vi "TestConfig.vi"(8 "error in":errorcluster {"code" format="Error %.0f"}, 11 "MainFGV_data":T1) -> (0 "error out":errorcluster {"code" format="Error %.0f"}, 3 "MainFGV_data out":T1)   [LabVIEW 2016]
uses:
  StrainGauge/SG_data.ctl
  CurrentMeter/CM_data.ctl
  CurrentMeter/CM_SerialNumber.ctl
  MainFGV_data.ctl
panel:
  in  "OK":bool
  in  "Cancelar":bool
  in  "OpenConfig":bool caption="Abrir\nconfiguração"
  in  "SaveConfig":bool caption="Salvar\nconfiguração"
  in  "CM_config":T2[](array[typedef])=[{"Serial"=enum."274124", "Coordenada X"=0.0, "Coordenada Y"=0.0, "ID"="CH 1", "active"=TRUE}, {"Serial"=enum."274125", "Coordenada X"=0.0, "Coordenada Y"=0.0, "ID"="CH 2", "active"=TRUE}, {"Serial"=enum."274126", "Coordenada X"=0.0, "Coordenada Y"=0.0, "ID"="CH 3", "active"=TRUE}, {"Serial"=enum."274127", "Coordenada X"=0.0, "Coordenada Y"=0.0, "ID"="CH 4", "active"=TRUE}, {"Serial"=enum."274128", "Coordenada X"=0.0, "Coordenada Y"=0.0, "ID"="CH 5", "active"=TRUE}]
  in  "SG_config":T4[](array[typedef])=[{"ID"="CH 1", "Sensibilidade"=2.0, "Descrição"="Extensômetro na grade", "active"=TRUE}, {"ID"="CH 2", "Sensibilidade"=2.0, "Descrição"="Extensômetro na grade", "active"=TRUE}, {"ID"="CH 3", "Sensibilidade"=2.0, "Descrição"="Extensômetro na grade", "active"=TRUE}, {"ID"="CH 4", "Sensibilidade"=2.0, "Descrição"="Extensômetro na grade", "active"=TRUE}, {"ID"="CH 5", "Sensibilidade"=2.0, "Descrição"="Extensômetro na grade", "active"=TRUE}, {"ID"="CH 6", "Sensibilidade"=2.0, "Descrição"="Extensômetro na grade", "active"=TRUE}, {"ID"="CH 7", "Sensibilidade"=2.0, "Descrição"="Extensômetro na grade", "active"=TRUE}, {"ID"="CH 8", "Sensibilidade"=2.0, "Descrição"="Extensômetro na grade", "active"=TRUE}, {"ID"="CH 9", "Sensibilidade"=2.0, "Descrição"="Extensômetro na grade", "active"=TRUE}, {"ID"="CH 10", "Sensibilidade"=2.0, "Descrição"="Extensômetro na grade", "active"=TRUE}, {"ID"="CH 11", "Sensibilidade"=2.0, "Descrição"="Extensômetro na grade", "active"=TRUE}, {"ID"="CH 12", "Sensibilidade"=2.0, "Descrição"="Extensômetro na grade", "active"=TRUE}, {"ID"="CH 13", "Sensibilidade"=2.0, "Descrição"="Extensômetro na grade", "active"=TRUE}, {"ID"="CH 14", "Sensibilidade"=2.0, "Descrição"="Extensômetro na grade", "active"=TRUE}, {"ID"="CH 15", "Sensibilidade"=2.0, "Descrição"="Extensômetro na grade", "active"=TRUE}, {"ID"="CH 16", "Sensibilidade"=2.0, "Descrição"="Extensômetro na grade", "active"=TRUE}, {"ID"="CH 17", "Sensibilidade"=2.0, "Descrição"="Extensômetro na grade", "active"=TRUE}, {"ID"="CH 18", "Sensibilidade"=2.0, "Descrição"="Extensômetro na grade", "active"=TRUE}, {"ID"="CH 19", "Sensibilidade"=2.0, "Descrição"="Extensômetro na grade", "active"=TRUE}, {"ID"="CH 20", "Sensibilidade"=2.0, "Descrição"="Extensômetro na grade", "active"=TRUE}, {"ID"="CH 21", "Sensibilidade"=2.0, "Descrição"="Extensômetro na grade", "active"=TRUE}, {"ID"="CH 22", "Sensibilidade"=2.0, "Descrição"="Extensômetro na grade", "active"=TRUE}, {"ID"="CH 23", "Sensibilidade"=2.0, "Descrição"="Extensômetro na grade", "active"=TRUE}, {"ID"="CH 24", "Sensibilidade"=2.0, "Descrição"="Extensômetro na grade", "active"=TRUE}]
  # "Extensômetros"
  # "Molinetes"
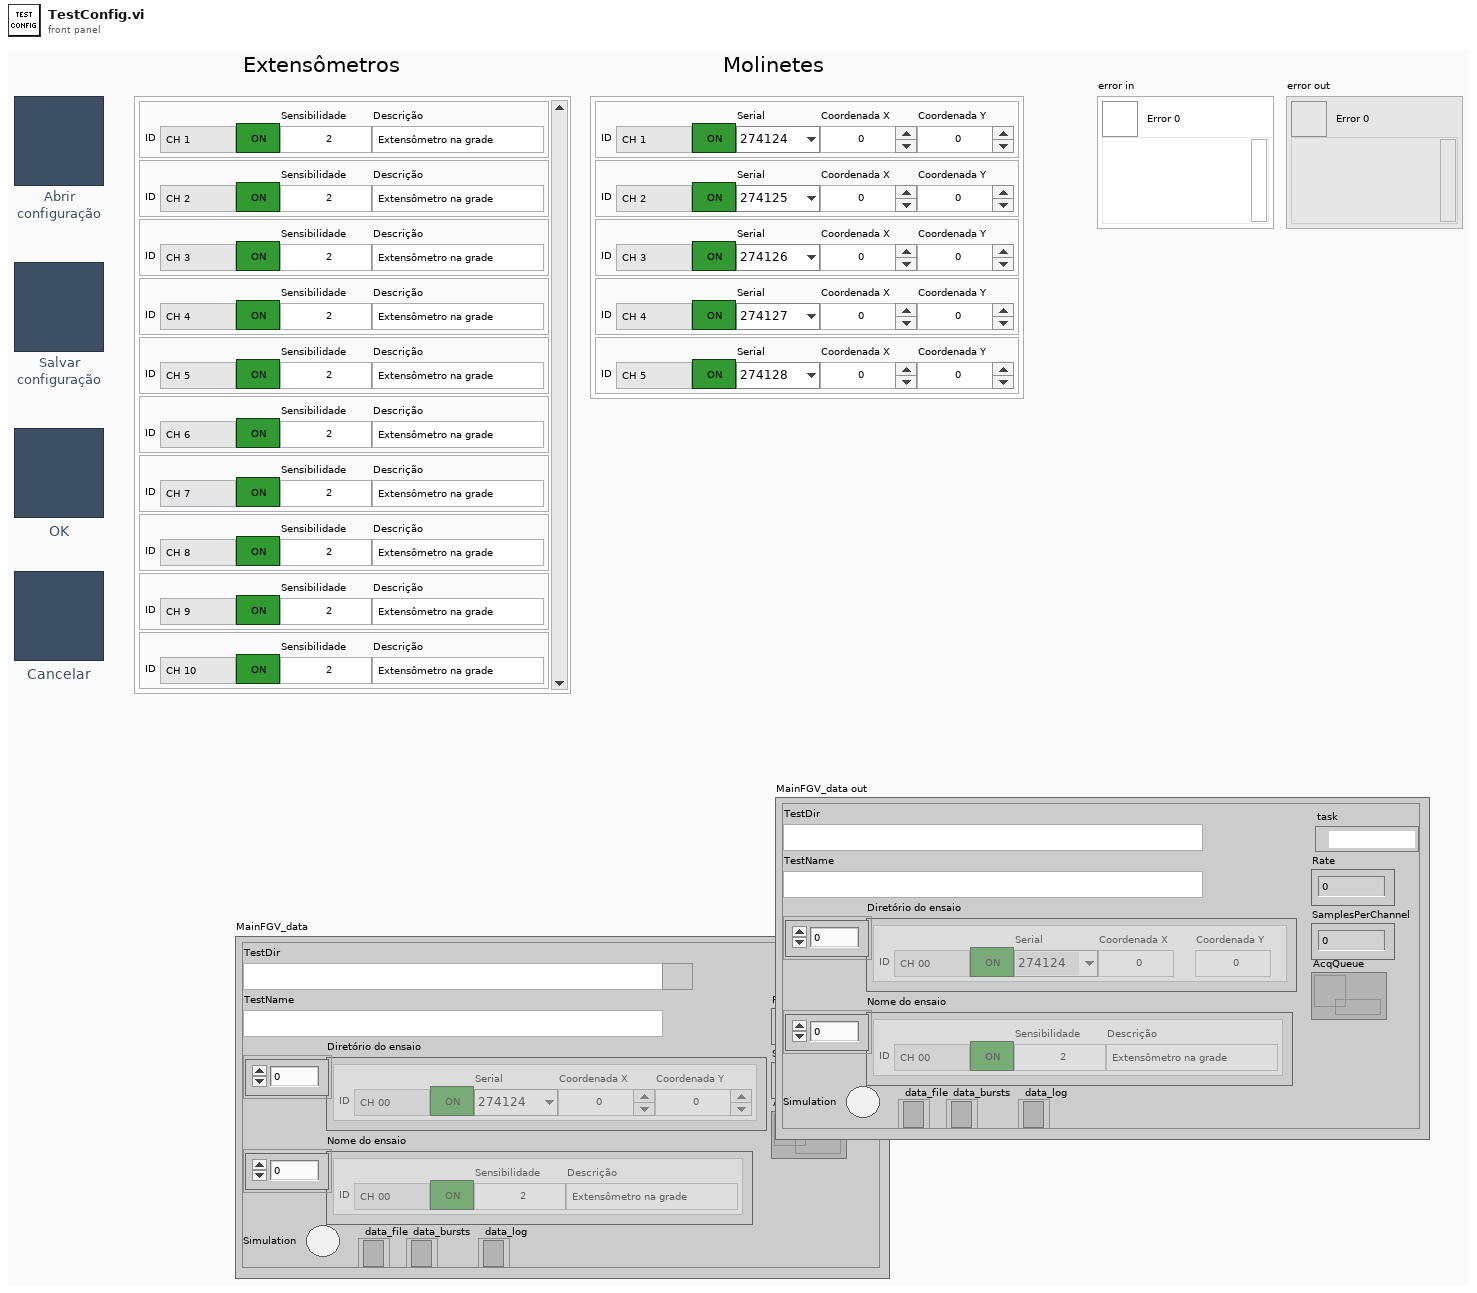
[diagram p1: front panel]
types:
  T1 = typedef "MainFGV_data.ctl" = cluster{"TestDir":path, "TestName":string, "CM_data":T2[], "SG_data":T4[], "Simulation":bool, "task":refnum<k21>, "data_file":refnum<file>, "data_bursts":refnum<file>, "data_log":refnum<file>, "Rate":dbl, "SamplesPerChannel":dbl, "AcqQueue":refnum<queue>}
  T2 = typedef "CM_data.ctl" = cluster{"Serial":T3, "Coordenada X":dbl, "Coordenada Y":dbl, "ID":string, "active":bool}
  T3 = typedef "CM_SerialNumber.ctl" = enum16{"274124", "274125", "274126", "274127", "274128"}
  T4 = typedef "SG_data.ctl" = cluster{"ID":string, "Sensibilidade":dbl, "Descrição":string, "active":bool}
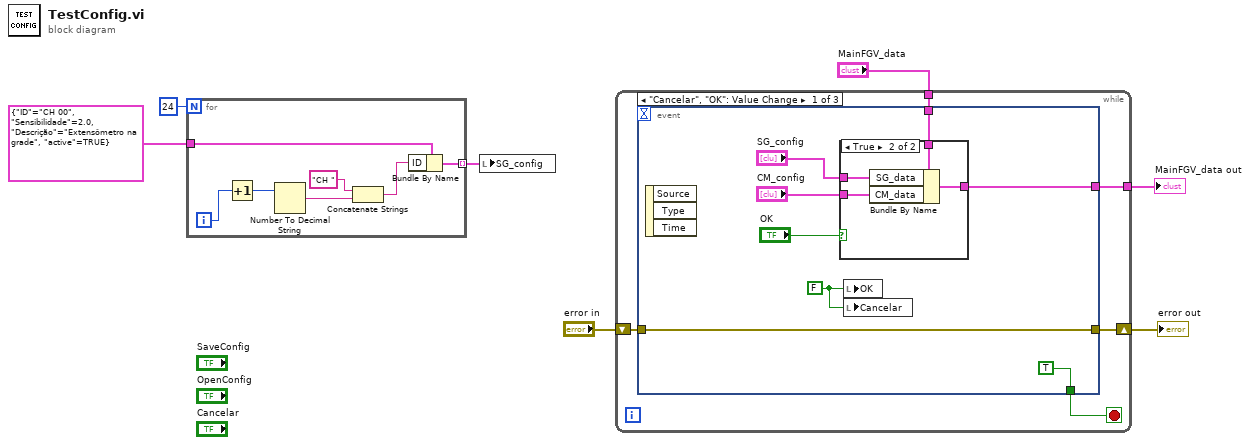
[diagram p0: block diagram]
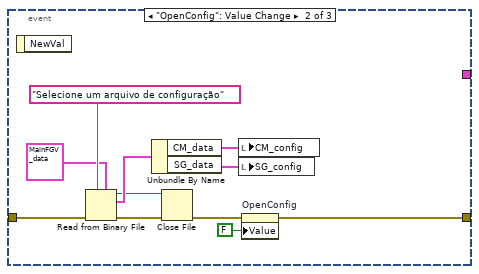
[diagram p3: hidden frame]
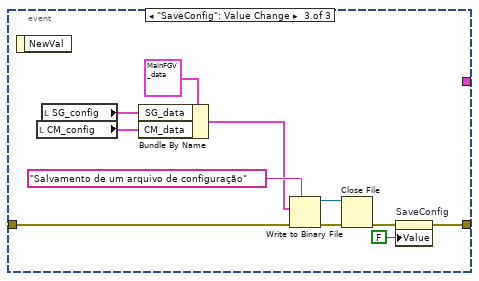
[diagram p4: hidden frame]
diagram:
  n1 = for {
    N: 24 -> [_]
    tunnel: T4 {"ID"="CH 00", "Sensibilidade"=2.0, "Descrição"="Extensômetro na grade", "active"=TRUE} ("StrainGauge_data") -> [w9]
    tunnel: [w8] -> w5 mode=indexing
    i -> [w14]
    n2 = Increment(x=w14) -> (x+1=w13:i32)
    n3 = Number To Decimal String(number=w13) -> (decimal integer string=w12:string)  [unwired: 1 in]
    n4 = Concatenate Strings("CH " ("string"), w12) -> (w10:string)
    n5 = Bundle By Name(cluster=w9, "ID"=w10) -> (w8:T4)
  }
  n6 = local write "SG_config"(w5) -> ()
  n7 = while {
    shift-right: [w17] -> w3
    shift-left: "error in" -> [w18]
    tunnel: "MainFGV_data" -> [w16]
    tunnel: [w15] -> w1
    stop <- w19 stop-if-true
    n8 = event shown="[0] \"Cancelar\", \"OK\": Value Change" {
      selector: _ -> [_ _ _]
      dyn-events: _ -> [_ _ _]
      timeout: _ -> [_ _ _]
      tunnel: [TRUE ("OK") _ _] -> w19
      tunnel: w18 -> [w26 w42 w50]
      tunnel: [w26 w33 w45] -> w17
      tunnel: w16 -> [w23 _ _]
      tunnel: [w22 _ _] -> w15
      event "Cancelar", "OK": Value Change {
        w21 = FALSE ("OK")
        n9 = event-data() -> ()  [unwired: 1 in, 3 out]
        n10 = case shown="True" "OK" {
          tunnel: "CM_config" -> [_ w32]
          tunnel: "SG_config" -> [_ w31]
          tunnel: w23 -> [w28 w30]
          tunnel: [w28 w29] -> w22
          frame False {
          }
          frame True {
            n11 = Bundle By Name(cluster=w30, "SG_data"=w31, "CM_data"=w32) -> (w29:T1)
          }
        }
        n12 = local write "OK"(w21) -> ()
        n13 = local write "Cancelar"(w21) -> ()
      }
      event "OpenConfig": Value Change {
        n14 = event-data() -> ()  [unwired: 1 in, 1 out]
        n15 = Read from Binary File(5:T1 {"TestDir"=path "C:/Users/l01481/Desktop/Teste_0", "TestName"="Teste", "CM_data"=[], "SG_data"=[], "Simulation"=TRUE, "task"="", "data_file"=refnum, "data_bursts"=refnum, "data_log"=refnum, "Rate"=0.0, "SamplesPerChannel"=0.0, "AcqQueue"=refnum} ("MainFGV_data"), 7:"Selecione um arquivo de configuração" ("prompt (Open existing file)"), 8:w42) -> (0:w39:errorcluster, 2:w40:T1, 3:w38:refnum<file>)  [unwired: 3 in, 1 out]
        n16 = Unbundle By Name(w40) -> ("CM_data"=w36:T2[], "SG_data"=w37:T4[])
        n17 = Close File(refnum=w38, error in=w39) -> (error out=w34:errorcluster)  [unwired: 1 out]
        n18 = local write "CM_config"(w36) -> ()
        n19 = local write "SG_config"(w37) -> ()
        n20 = property on="OpenConfig" class="Bool (strict)"(error in=w34, "Value"=FALSE ("SaveConfig")) -> (error out=w33:errorcluster)  [unwired: 1 in, 1 out]
      }
      event "SaveConfig": Value Change {
        n21 = event-data() -> ()  [unwired: 1 in, 1 out]
        n22 = local read "CM_config"() -> (w52:T2[])
        n23 = local read "SG_config"() -> (w53:T4[])
        n24 = Bundle By Name(cluster=T1 {"TestDir"=path "C:/Users/l01481/Desktop/Teste_0", "TestName"="Teste", "CM_data"=[], "SG_data"=[], "Simulation"=TRUE, "task"="", "data_file"=refnum, "data_bursts"=refnum, "data_log"=refnum, "Rate"=0.0, "SamplesPerChannel"=0.0, "AcqQueue"=refnum} ("MainFGV_data"), "SG_data"=w53, "CM_data"=w52) -> (w47:T1)
        n25 = Write to Binary File(data=w47, error in=w50, 7:"Salvamento de um arquivo de configuração" ("prompt (Choose or enter file path)")) -> (refnum out=w48:refnum<file>, error out=w49:errorcluster)  [unwired: 3 in, 1 out]
        n26 = Close File(refnum=w48, error in=w49) -> (error out=w46:errorcluster)  [unwired: 1 out]
        n27 = property on="SaveConfig" class="Bool (strict)"(error in=w46, "Value"=FALSE ("SaveConfig")) -> (error out=w45:errorcluster)  [unwired: 1 in, 1 out]
      }
    }
  }
  "MainFGV_data out" <- w1
  "error out" <- w3
